vi "CFN61G_U8-to-B87-90_v1.vi"(11 "U8_Input":u8[](array[numeric])) -> (2 "Align_Word":u16(slide) scale=0.0..65535.0, 3 "Op_Word":u16(slide) scale=0.0..65535.0)   [LabVIEW 2017]
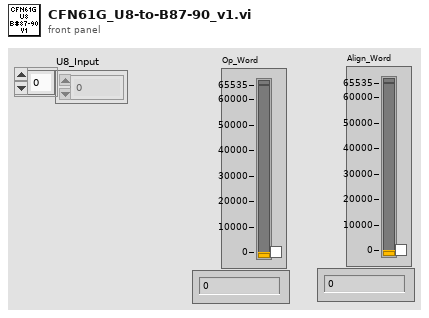
[diagram p1: front panel]
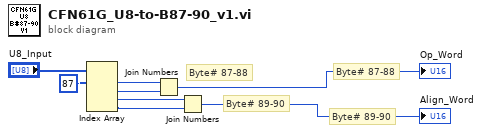
[diagram p0: block diagram]
diagram:
  # "Byte# 89-90"
  # "Byte# 87-88"
  # "Byte# 89-90"
  # "Byte# 87-88"
  n1 = Index Array(array="U8_Input", index #1=87 ("index")) -> (element #1=w5:u8, element #2=w6:u8, element #3=w7:u8, element #4=w8:u8)  [unwired: 3 in]
  n2 = Join Numbers(hi=w5, lo=w6) -> ((hi.lo)=→"Op_Word":u16)
  n3 = Join Numbers(hi=w7, lo=w8) -> ((hi.lo)=→"Align_Word":u16)
